vi "Build Array (Single).vi"(8 "error in (no error)":errorcluster, 10 "JSON Datatype":refnum<class "JSON Datatype.lvclass">, 11 "JSON Array in":refnum<class "JSON Array.lvclass">) -> (0 "error out":errorcluster, 3 "JSON Array out":refnum<class "JSON Array.lvclass">)   [LabVIEW 2017, in "LVJSON.lvlib" / "JSON Array.lvclass"]
uses:
  JSON Array.lvclass
  JSON Datatype/JSON Datatype.lvclass
  JSON Array.lvclass/JSON Array.ctl
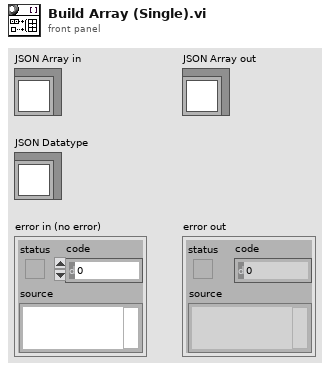
[diagram p1: front panel]
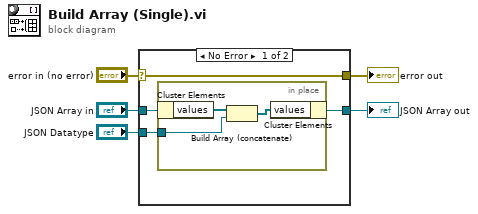
[diagram p0: block diagram]
diagram:
  n1 = case shown="No Error" "error in (no error)" {
    selector: "error in (no error)" -> [w9 w14]
    tunnel: [w9 w14] -> w4
    tunnel: [w6 w13] -> w2
    tunnel: "JSON Array in" -> [w8 w13]
    tunnel: "JSON Datatype" -> [w7 _]
    frame No Error {
      n2 = in-place {
        in-place-border: w7 -> [w11]
        n3 = in-place-cluster #1(w8) -> ("values"=w10:refnum<class "JSON Datatype.lvclass">[])
        n4 = Build Array (concatenate)(w10, w11) -> (w12:refnum<class "JSON Datatype.lvclass">[])
        n5 = in-place-cluster #1("values"=w12) -> (w6:refnum<class "JSON Array.lvclass">)
      }
    }
    frame Error {
    }
  }
  "error out" <- w4
  "JSON Array out" <- w2
